vi "CAENHV Set Bd Param Bitfield.vi"(7 "ParValue":bool[](array[boolean]), 8 "error in (no error)":errorcluster, 9 "ParName":string, 10 "slot":u16, 11 "handle":i32) -> (0 "error out":errorcluster)   [LabVIEW 2018, in "CAENHVWrapper.lvlib"]
doc: "CAENHVLIB_API CAENHVRESULT CAENHV_SetBdParam(int handle, \n ushort slotNum, const ushort *slotList, const char *ParName, void *ParValue);"
uses:
  <instrlib>/CAENHVWrapper/CAENHVWrapper.lvlib
  <instrlib>/CAENHVWrapper/VIs/CAENHVWrapper.dll
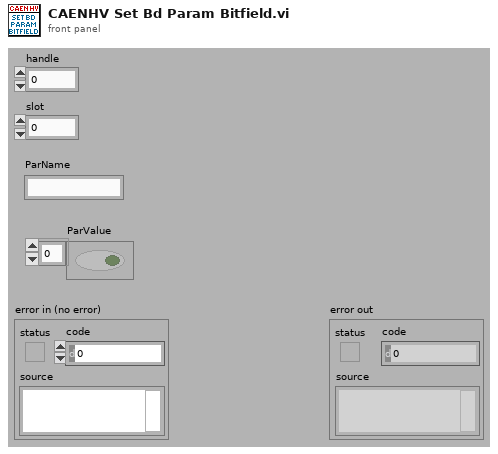
[diagram p1: front panel]
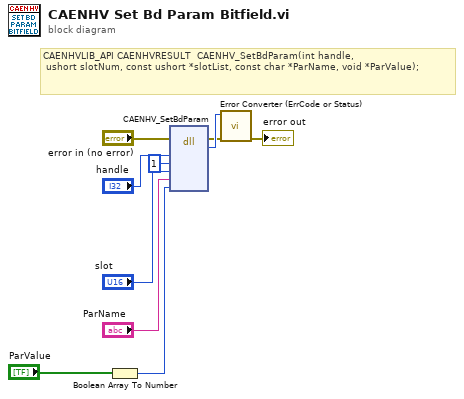
[diagram p0: block diagram]
diagram:
  # "CAENHVLIB_API CAENHVRESULT  CAENHV_SetBdParam(int handle, \n ushort slotNum, const ushort *slotList, const char *ParName, void *ParValue);"
  n1 = Boolean Array To Number(Boolean array="ParValue") -> (number=w3:u32)
  n2 = dll-call lib="C:/Program Files (x86)/National Instruments/LabVIEW 2018/instr.lib/CAENHVWrapper/VIs/CAENHVWrapper.*" fn="CAENHV_SetBdParam"(error in="error in (no error)", "handle"="handle", "slotNum"=u16 1, "slotList"="slot", "ParName"="ParName", "ParValue"=w3) -> (error out=w5:errorcluster, "return type"=w6:i32)  [unwired: 7 in, 1 out]
  n3 = call <instrlib>:"Error Converter (ErrCode or Status).vi"("error in (no error)"=w5, "error code"=w6) -> ("error out"=→"error out":errorcluster)  [unwired: 9 in]
